vi "Convert to String (Local Decimal).vi"(11 "Distance (String)":string) -> (3 "Distance (DBL)":dbl)   [LabVIEW 2024]
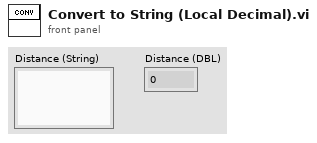
[diagram p1: front panel]
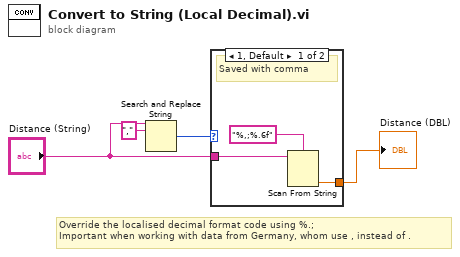
[diagram p0: block diagram]
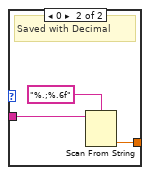
[diagram p2: hidden frame]
diagram:
  # "Override the localised decimal format code using %.;\nImportant when working with data from Germany, whom use , instead of ."
  n1 = Search and Replace String(input string="Distance (String)", search string=",") -> (number of replacements=w1:i32)  [unwired: 6 in, 3 out]
  n2 = case shown="1, Default" w1 {
    tunnel: "Distance (String)" -> [w7 w10]
    tunnel: [w5 w8] -> w4
    frame 1, Default {
      # "Saved with comma"
      n3 = Scan From String(format string="%,;%.6f", input string=w7) -> (output 1=w5:dbl)  [unwired: 3 in, 3 out]
    }
    frame 0 {
      # "Saved with Decimal"
      n4 = Scan From String(format string="%.;%.6f", input string=w10) -> (output 1=w8:dbl)  [unwired: 3 in, 3 out]
    }
  }
  "Distance (DBL)" <- w4
